vi "Find Neighbour Points (SubVI).vi"(8 "Previous HT Position":u64, 11 "Current HT Position":u64) -> (0 "Increment Vote":bool, 3 "Neighbor Point":u64)   [LabVIEW 2020]
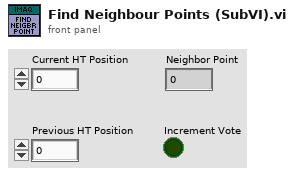
[diagram p1: front panel]
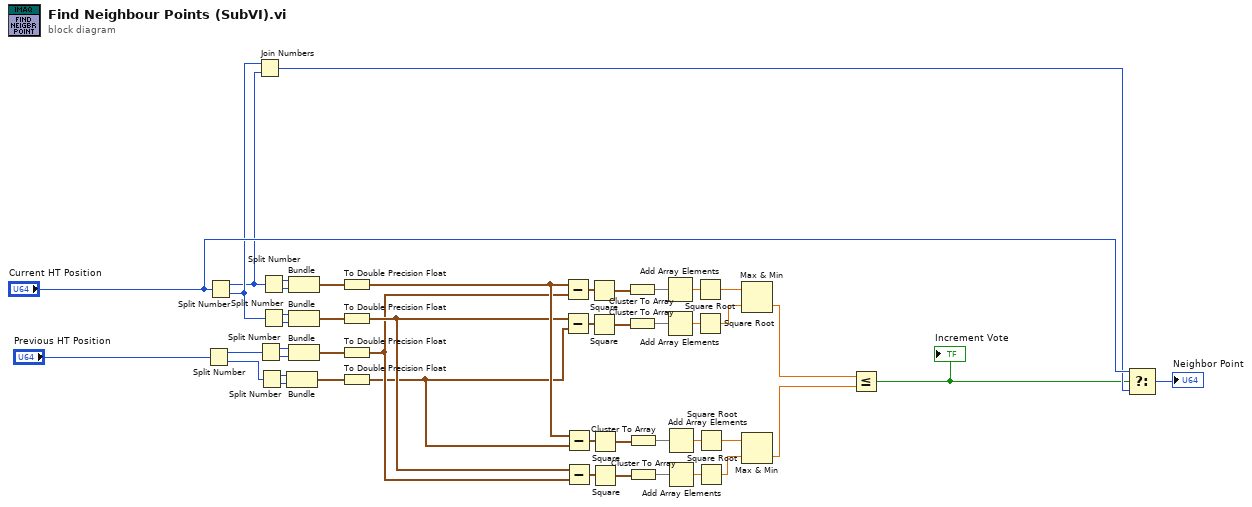
[diagram p0: block diagram]
diagram:
  n1 = Split Number(x="Previous HT Position") -> (hi(x)=w36:u32, lo(x)=w37:u32)
  n2 = Split Number(x="Current HT Position") -> (hi(x)=w17:u32, lo(x)=w18:u32)
  n3 = Join Numbers(hi=w18, lo=w17) -> ((hi.lo)=w16:u64)
  n4 = Split Number(x=w36) -> (hi(x)=w39:u16, lo(x)=w38:u16)
  n5 = Split Number(x=w37) -> (hi(x)=w41:u16, lo(x)=w40:u16)
  n6 = Split Number(x=w17) -> (hi(x)=w44:u16, lo(x)=w45:u16)
  n7 = Split Number(x=w18) -> (hi(x)=w42:u16, lo(x)=w43:u16)
  n8 = Bundle(w41, w40) -> (w3:cluster{u16, u16})  [unwired: 1 in]
  n9 = Bundle(w44, w45) -> (w8:cluster{u16, u16})  [unwired: 1 in]
  n10 = Bundle(w42, w43) -> (w6:cluster{u16, u16})  [unwired: 1 in]
  n11 = Bundle(w39, w38) -> (w4:cluster{u16, u16})  [unwired: 1 in]
  n12 = To Double Precision Float(number=w8) -> (double precision float=w7:cluster{dbl, dbl})
  n13 = To Double Precision Float(number=w6) -> (double precision float=w5:cluster{dbl, dbl})
  n14 = To Double Precision Float(number=w4) -> (double precision float=w2:cluster{dbl, dbl})
  n15 = To Double Precision Float(number=w3) -> (double precision float=w1:cluster{dbl, dbl})
  n16 = Subtract(x=w7, y=w2) -> (x-y=w27:cluster{dbl, dbl})
  n17 = Subtract(x=w5, y=w1) -> (x-y=w30:cluster{dbl, dbl})
  n18 = Subtract(x=w7, y=w1) -> (x-y=w26:cluster{dbl, dbl})
  n19 = Subtract(x=w5, y=w2) -> (x-y=w23:cluster{dbl, dbl})
  n20 = Square(x=w27) -> (x^2=w46:cluster{dbl, dbl})
  n21 = Square(x=w30) -> (x^2=w29:cluster{dbl, dbl})
  n22 = Square(x=w26) -> (x^2=w20:cluster{dbl, dbl})
  n23 = Square(x=w23) -> (x^2=w24:cluster{dbl, dbl})
  n24 = Cluster To Array(cluster=w46) -> (array=w32:dbl[])
  n25 = Cluster To Array(cluster=w29) -> (array=w31:dbl[])
  n26 = Cluster To Array(cluster=w20) -> (array=w21:dbl[])
  n27 = Cluster To Array(cluster=w24) -> (array=w22:dbl[])
  n28 = Add Array Elements(numeric array=w32) -> (sum=w47:dbl)
  n29 = Add Array Elements(numeric array=w31) -> (sum=w28:dbl)
  n30 = Add Array Elements(numeric array=w21) -> (sum=w19:dbl)
  n31 = Add Array Elements(numeric array=w22) -> (sum=w25:dbl)
  n32 = Square Root(x=w47) -> (sqrt(x)=w15:dbl)
  n33 = Square Root(x=w28) -> (sqrt(x)=w14:dbl)
  n34 = Square Root(x=w19) -> (sqrt(x)=w13:dbl)
  n35 = Square Root(x=w25) -> (sqrt(x)=w12:dbl)
  n36 = Max & Min(x=w15, y=w14) -> (min(x,y)=w11:dbl)  [unwired: 1 out]
  n37 = Max & Min(x=w13, y=w12) -> (min(x,y)=w10:dbl)  [unwired: 1 out]
  n38 = Less Or Equal?(x=w11, y=w10) -> (x <= y?=w9:bool)
  "Increment Vote" <- w9
  n39 = Select(t="Current HT Position", s=w9, f=w16) -> (s? t:f=→"Neighbor Point":u64)
